vi "Acknowldge Quench.vi"(7 "Address":u16, 8 "Error In":errorcluster, 11 "VISA Resource in":refnum<visa-resource-name>) -> (0 "Error Out":errorcluster, 3 "VISA Resource out":refnum<visa-resource-name>)   [LabVIEW 2014, in "KIT QV.lvlib"]
doc: "Acknowledge quench.\n\n<b>Attention:</b> If the quench condition still exists, the error : Command not executable will be returned. This happens to avoid dataloss."
uses:
  KIT QV.lvlib
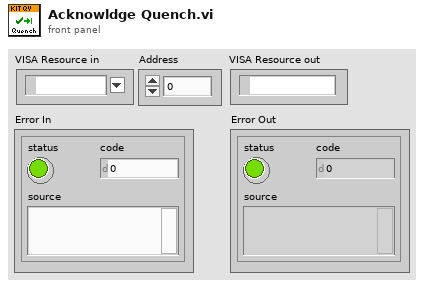
[diagram p1: front panel]
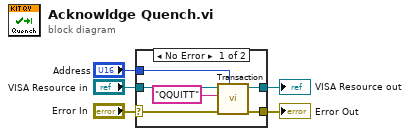
[diagram p0: block diagram]
diagram:
  n1 = case shown="No Error" "Error In" {
    selector: "Error In" -> [w10 w12]
    tunnel: [w7 w13] -> w5
    tunnel: [w6 w12] -> w4
    tunnel: "VISA Resource in" -> [w11 w13]
    tunnel: "Address" -> [w8 _]
    frame No Error {
      n2 = call "Transaction.vi"("Address"=w8, "error in (no error)"=w10, "Command"="QQUITT" ("Reset Command"), "VISA Resource in"=w11) -> ("error out"=w6:errorcluster, "VISA Resource out"=w7:refnum<visa-resource-name>)  [unwired: 5 in, 1 out]
    }
    frame Error {
    }
  }
  "Error Out" <- w4
  "VISA Resource out" <- w5
